vi "hPa_to_inHg.vi"(1 "hPa":sgl) -> (0 "inHg":sgl)   [LabVIEW 2012]
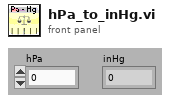
[diagram p1: front panel]
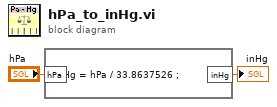
[diagram p0: block diagram]
diagram:
  n1 = formula code="inHg = hPa / 33.8637526 ;"("hPa"="hPa") -> ("inHg"=→"inHg":dbl)
